vi "ShutdownEvent.vi"(8 "ErrorArray":errorcluster[](array[cluster])) -> (0 "ErrorArray":errorcluster[](array[cluster]))   [LabVIEW 2018]
uses:
  clUserEventDataType.ctl
  <vilib>/event_ctls.llb/usereventprio.ctl
  <userlib>/NIST/NISTErrorLib/NISTErrorLib.lvlib
  NistPluggableModules/Visualization/VisualizeBase/VisualizeBase_class/VisualizeBase.lvclass
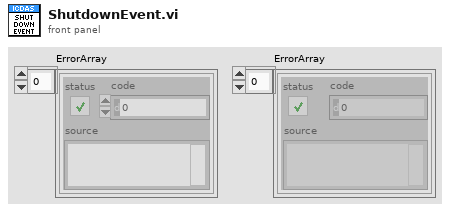
[diagram p1: front panel]
types:
  T1 = typedef "usereventprio.ctl" = enum32{"high priority", "normal priority"}
  T2 = typedef "clUserEventDataType.ctl" = cluster{"Data":variant}
  T3 = typedef "ICDASUserEvents.ctl" = cluster{"StopEvent":refnum<user-event>, "RefreshUserEvents":refnum<user-event>, "StatusUpdate":refnum<user-event>, "RunAllScripts":refnum<user-event>, "ShutdownEvent":refnum<user-event>, "TestMgrDidStop":refnum<user-event>, "PluginMgrDidStop":refnum<user-event>}
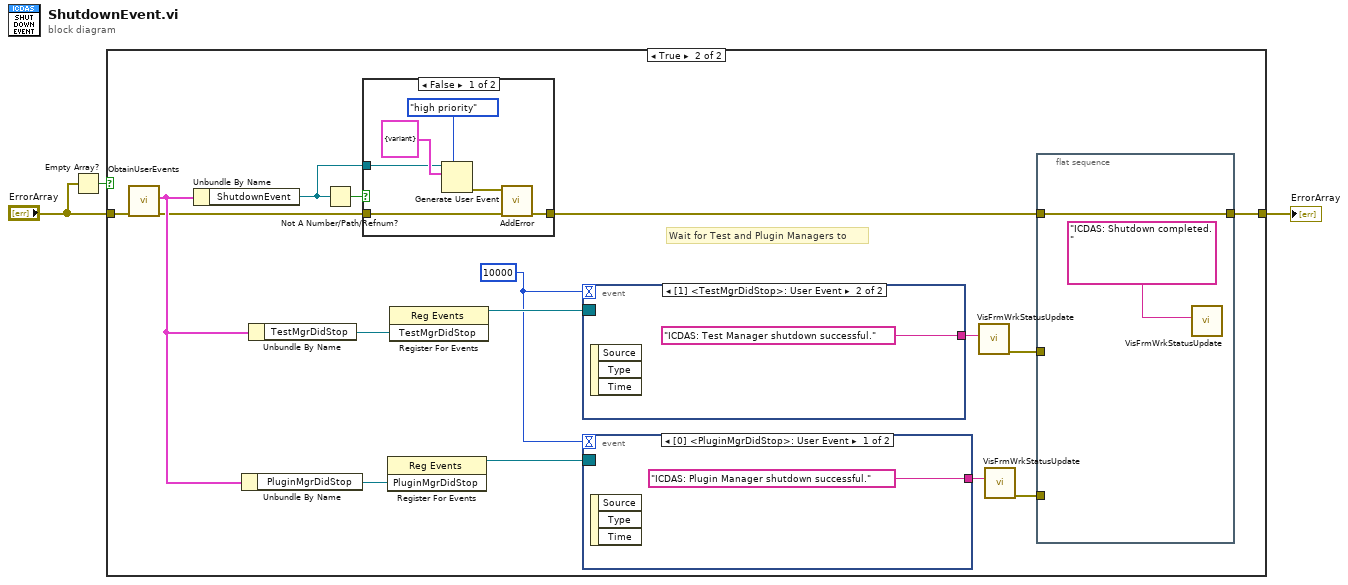
[diagram p0: block diagram]
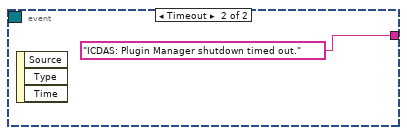
[diagram p3: hidden frame]
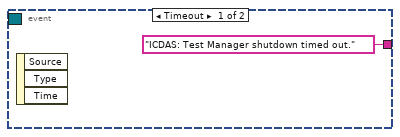
[diagram p4: hidden frame]
diagram:
  n1 = Empty Array?(array="ErrorArray") -> (empty?=w3:bool)
  n2 = case shown="True" w3 {
    tunnel: "ErrorArray" -> [w4 w18]
    tunnel: [w4 w12] -> w1
    frame False {
    }
    frame True {
      w8 = 10000
      # "Wait for Test and Plugin Managers to"
      n3 = call "ObtainUserEvents.vi"("ErrorArray"=w18) -> ("ErrorArray"=w11:errorcluster[], "ICDASUserEvents"=w15:T3)  [unwired: 9 in]
      n4 = Unbundle By Name(w15) -> ("ShutdownEvent"=w19:refnum<user-event>)
      n5 = Unbundle By Name(w15) -> ("PluginMgrDidStop"=w5:refnum<user-event>)
      n6 = Unbundle By Name(w15) -> ("TestMgrDidStop"=w6:refnum<user-event>)
      n7 = Not A Number/Path/Refnum?(number/path/refnum=w19) -> (NaN/Path/Refnum?=w20:bool)
      n8 = case shown="False" w20 {
        tunnel: w11 -> [w30 w33]
        tunnel: w19 -> [w31 _]
        tunnel: [w27 w33] -> w7
        frame False {
          n9 = Generate User Event(priority (normal)=usereventprio."high priority", user event=w31, event data cluster=T2 {"Data"=variant} ("clUserEventData")) -> (error out=w29:errorcluster)  [unwired: 1 in, 1 out]
          n10 = call <userlib>:"AddError.vi"("ErrorArray In"=w30, "error in (no error)"=w29) -> ("ErrorArray Out"=w27:errorcluster[])  [unwired: 8 in, 1 out]
        }
        frame True {
        }
      }
      n11 = register-events(w5) -> (reference out=w17:refnum<event-registration>)  [unwired: 2 in, 1 out]
      n12 = register-events(w6) -> (reference out=w16:refnum<event-registration>)  [unwired: 2 in, 1 out]
      n13 = event shown="[1] <TestMgrDidStop>: User Event" {
        selector: w16 -> [_ _]
        dyn-events: _ -> [_ _]
        timeout: w8 -> [_ _]
        tunnel: ["ICDAS: Test Manager shutdown timed out." ("Status") "ICDAS: Test Manager shutdown successful." ("Status")] -> w14
        event Timeout {
          n14 = event-data() -> ()  [unwired: 1 in, 3 out]
        }
        event User Event {
          n15 = event-data() -> ()  [unwired: 1 in, 3 out]
        }
      }
      n16 = event shown="[0] <PluginMgrDidStop>: User Event" {
        selector: w17 -> [_ _]
        dyn-events: _ -> [_ _]
        timeout: w8 -> [_ _]
        tunnel: ["ICDAS: Plugin Manager shutdown successful." ("Status") "ICDAS: Plugin Manager shutdown timed out." ("Status")] -> w13
        event User Event {
          n17 = event-data() -> ()  [unwired: 1 in, 3 out]
        }
        event Timeout {
          n18 = event-data() -> ()  [unwired: 1 in, 3 out]
        }
      }
      n19 = call "VisFrmWrkStatusUpdate.vi"("Status"=w14) -> ("error out"=w10:errorcluster)  [unwired: 10 in]
      n20 = call "VisFrmWrkStatusUpdate.vi"("Status"=w13) -> ("error out"=w9:errorcluster)  [unwired: 10 in]
      n21 = flat-sequence {
        tunnel: [w21] -> w12
        tunnel: w7 -> [w21]
        tunnel: w10 -> [_]
        tunnel: w9 -> [_]
        frame #0 {
          n22 = call "VisFrmWrkStatusUpdate.vi"("Status"="ICDAS: Shutdown completed.") -> ()  [unwired: 10 in, 1 out]
        }
      }
    }
  }
  "ErrorArray" <- w1
